vi "configure.vi"(8 "error in (no error)":errorcluster, 10 "SerialConfig":T1={"VISA resource name"="", "Baud Rate"=9600, "Data Bits"=8, "Parity"=enum."None", "Stop Bits"=10, "Flow Control"=0, "Timeout (ms)"=10000, "Serial Protocol"=enum."RS485"} {"Stop Bits" items=["1.0"=10, "1.5"=15, "2.0"=20]; "Flow Control" items=["None", "XON/XOFF", "RTS/CTS", "XON/XOFF & RTS/CTS", "DTR/DSR", "XON/XOFF & DTR/DSR"]; "Data Bits" min=5 max=8 step=1}, 11 "SerialReal in":refnum<class "SerialReal.lvclass">) -> (0 "error out":errorcluster, 3 "SerialReal out":refnum<class "SerialReal.lvclass">)   [LabVIEW 2013, in "SerialProtocols.lvlib" / "SerialReal.lvclass"]
uses:
  <userlib>/Common/SerialProtocols/SerialCommunicator/SerialReal/SerialReal.lvclass
  <userlib>/Common/SerialProtocols/Configuration/SerialConfig.ctl
  <userlib>/Common/SerialProtocols/Configuration/SerialProtocol.ctl
  <userlib>/Common/SerialProtocols/SerialCommunicator/SerialReal/SerialReal.lvclass/SerialReal.ctl
  <vilib>/Instr/_visa.llb/VISA Configure Serial Port (Instr).vi
  <userlib>/Common/SerialProtocols/SerialProtocols.lvlib
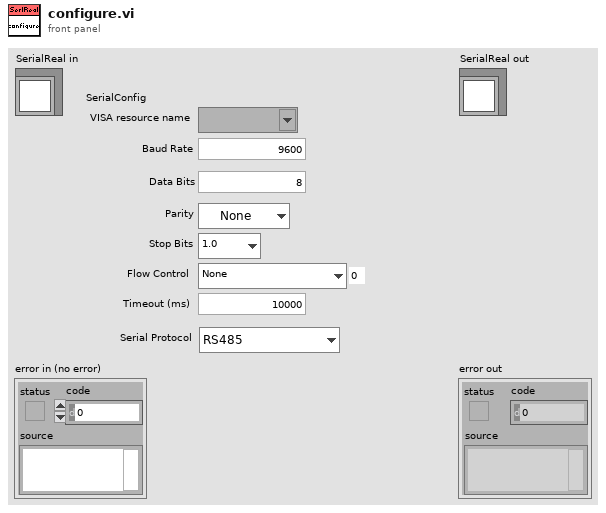
[diagram p1: front panel]
types:
  T1 = typedef "SerialProtocols.lvlib/SerialConfig.ctl" = cluster{"VISA resource name":refnum<visa-resource-name>, "Baud Rate":u32, "Data Bits":u16, "Parity":enum16{"None", "Odd", "Even", "Mark", "Space"}, "Stop Bits":u16, "Flow Control":u16, "Timeout (ms)":u32, "Serial Protocol":T2}
  T2 = typedef "SerialProtocols.lvlib/SerialProtocol.ctl" = enum16{"RS232", "RS485", "SerialSimulator"}
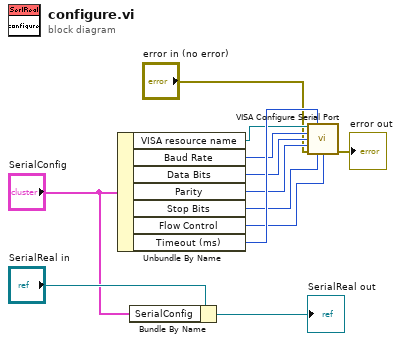
[diagram p0: block diagram]
diagram:
  n1 = Unbundle By Name("SerialConfig") -> ("VISA resource name"=w11:refnum<visa-resource-name>, "Baud Rate"=w10:u32, "Data Bits"=w9:u16, "Parity"=w8:enum16{"None", "Odd", "Even", "Mark", "Space"}, "Stop Bits"=w7:u16, "Flow Control"=w6:u16, "Timeout (ms)"=w12:u32)
  n2 = Bundle By Name(cluster="SerialReal in", "SerialConfig"="SerialConfig") -> (→"SerialReal out":refnum<class "SerialReal.lvclass">)
  n3 = call-poly "VISA Configure Serial Port"("VISA resource name"=w11, "timeout (10sec)"=w12, "baud rate (9600)"=w10, "data bits (8)"=w9, "parity (0:none)"=w8, "error in (no error)"="error in (no error)", "stop bits (10: 1 bit)"=w7, "flow control (0:none)"=w6) -> ("error out"=→"error out":errorcluster)  [unwired: 6 in, 1 out]
